vi "Teleop.vi"(10 "Match Info":T2={"Autonomous Elapsed Seconds"=0.0, "TeleOp Elapsed Seconds"=0.0, "Disabled Elapsed Seconds"=0.0, "Visited Autonomous"=FALSE, "Visited TeleOp"=FALSE, "Visited Disabled"=FALSE, "Autonomous Settings"={"Autonomous Style"=enum."Independent", "VI Refnum"=refnum}}, 11 "Call Context":T3) -> ()   [LabVIEW 2020]
doc: "This VI is called for each TeleOp packet received from the DS where the robot is not disabled. It is often used to read from the joysticks and update I/O or to update setpoints for timed control loops. It should complete and return within 20 milliseconds or it may miss DS packets."
uses:
  <vilib>/Rock Robotics/WPI/DriverStation/WPI_DriverStationDerivedRobotMode.ctl
  <vilib>/Rock Robotics/WPI/DriverStation/WPI_DriverStationMatch Info.ctl
  <vilib>/Rock Robotics/WPI/ThirdParty/Phoenix-LabVIEW/Motor Controller/Controls/CTRE_Phoenix_MotorControl_ControlMode.ctl
  <vilib>/Rock Robotics/Network Tables/NT Read Boolean.vi
  <vilib>/Rock Robotics/Network Tables/NT Read Number.vi
  <vilib>/Rock Robotics/WPI/ThirdParty/Phoenix-LabVIEW/CANCoder/Get/CTRE_Phoenix_CANcoder_GetSensorData.vi
  <vilib>/Rock Robotics/WPI/Utilities/WPI_GetSetVariantRefNum.vi
  <vilib>/addons/control/pid/pid.llb/PID (DBL).vi
  <vilib>/addons/control/pid/NI_PID_pid.lvlib
panel:
  in  "ScaleSpeed 4":dbl
  in  "ScaleSpeed 3":dbl
  in  "ScaleSpeed 2":dbl
  in  "ScaleSpeed":dbl
  in  "PID gains 2":T1={"proportional gain (Kc)"=0.002, "integral time (Ti, min)"=0.01, "derivative time (Td, min)"=0.0} {"derivative time (Td, min)" format="%.3f"; "integral time (Ti, min)" format="%.4f"; "proportional gain (Kc)" format="%.3f"}
  out "atan2(y,x)":dbl
  out "Absolute Position BL":dbl
  out "Absolute Position BR":dbl
  out "Absolute Position FL":dbl
  out "Absolute Position FR":dbl
  in  "PID gains":T1={"proportional gain (Kc)"=0.002, "integral time (Ti, min)"=0.01, "derivative time (Td, min)"=0.0} {"derivative time (Td, min)" format="%.3f"; "integral time (Ti, min)" format="%.4f"; "proportional gain (Kc)" format="%.3f"}
  in  "Output":dbl(knob) scale=-180.0..180.0
  out "Sample Slider 0":dbl(slide) scale=0.0..5.0
  out "Sample Boolean 1":bool
  out "Sample Boolean 0":bool
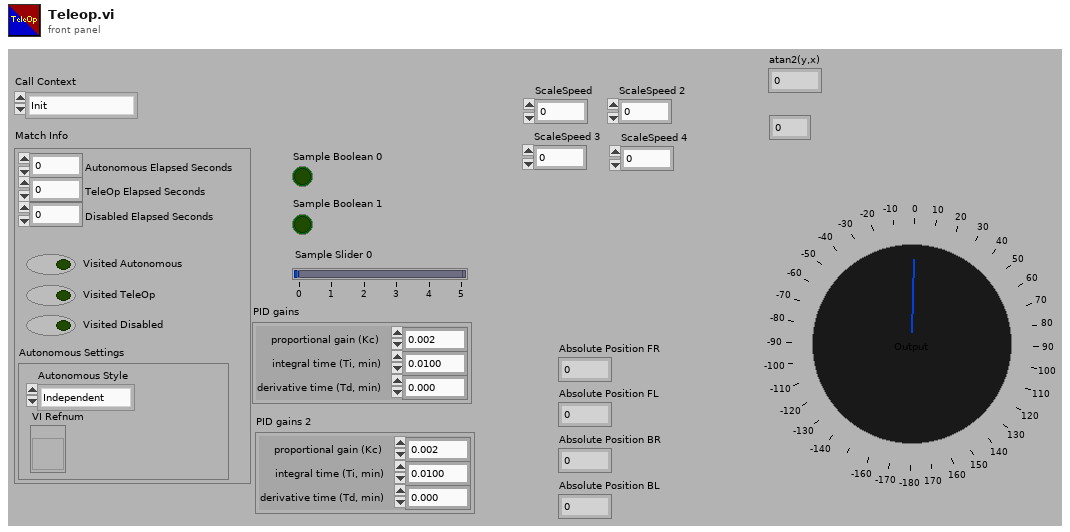
[diagram p1: front panel]
types:
  T1 = cluster{"proportional gain (Kc)":dbl, "integral time (Ti, min)":dbl, "derivative time (Td, min)":dbl}
  T2 = typedef "WPI_DriverStationMatch Info.ctl" = cluster{"Autonomous Elapsed Seconds":dbl, "TeleOp Elapsed Seconds":dbl, "Disabled Elapsed Seconds":dbl, "Visited Autonomous":bool, "Visited TeleOp":bool, "Visited Disabled":bool, "Autonomous Settings":cluster{"Autonomous Style":enum16{"Iterative", "Independent"}, "VI Refnum":refnum<vi>}}
  T3 = typedef "WPI_DriverStationDerivedRobotMode.ctl" = enum16{"Init", "Execute", "Stop"}
  T4 = typedef "CTRE_Phoenix_MotorControl_ControlMode.ctl" = u16
  T5 = typedef "CTRE_Phoenix_CANcoder_DeviceRef.ctl" = cluster{"DeviceStatus":errorcluster, "Device Number":u8, "Handle":u64, "UsageFrame":u32, "Library Path":path}
  T6 = typedef "WPI_JoystickDevRef.ctl" = cluster{"Device":T7}
  T7 = typedef "WPI_JoystickDeviceEnum.ctl" = enum16{"USB 0", "USB 1", "USB 2", "USB 3", "USB 4", "USB 5"}
  T8 = typedef "WPI_MotorControlDeviceRef.ctl" = cluster{"DeviceStatus":errorcluster, "Type":T9, "PWM":cluster{"PWM Channel":T10, "DeadBand":T11}, "CAN":cluster{"Device Number":u8, "SetOutput VI Ref":variant, "GetOutput VI Ref":variant, "Enable VI Ref":variant, "Disable VI Ref":variant, "Data":variant}, "Invert":bool, "DIO PWM":cluster{"PWM \"Enable\" Channel":T10, "DIOChannel":T12, "PWM Rate":dbl}}
  T9 = typedef "WPI_MotorControlType.ctl" = enum16{"PWM", "CAN", "DIO PWM"}
  T10 = typedef "FPGA_DIOPWMChannel.ctl" = enum8{"PWM 0", "PWM 1", "PWM 2", "PWM 3", "PWM 4", "PWM 5", "PWM 6", "PWM 7", "PWM 8", "PWM 9", "PWM MXP 0", "PWM MXP 1", "PWM MXP 2", "PWM MXP 3", "PWM MXP 4", "PWM MXP 5", "PWM MXP 6", "PWM MXP 7", "PWM MXP 8", "PWM MXP 9", "Invalid"}
  T11 = typedef "WPI_PWMDeadband.ctl" = cluster{"Name":string, "maxPositivePwm":i32, "minPositivePwm":i32, "centerPwm":i32, "maxNegativePwm":i32, "minNegativePwm":i32, "angularRange":u16}
  T12 = typedef "FPGA_DIOChannel.ctl" = enum8{"DIO 0", "DIO 1", "DIO 2", "DIO 3", "DIO 4", "DIO 5", "DIO 6", "DIO 7", "DIO 8", "DIO 9", "DIO MXP 0", "DIO MXP 1", "DIO MXP 2", "DIO MXP 3", "DIO MXP 4", "DIO MXP 5", "DIO MXP 6", "DIO MXP 7", "DIO MXP 8", "DIO MXP 9", "DIO MXP 10", "DIO MXP 11", "DIO MXP 12", "DIO MXP 13", "DIO MXP 14", "DIO MXP 15", "SPI Port CS1", "SPI Port CS2", "SPI Port CS3", "SPI Port MISO", "SPI Port MOSI", "Invalid"}
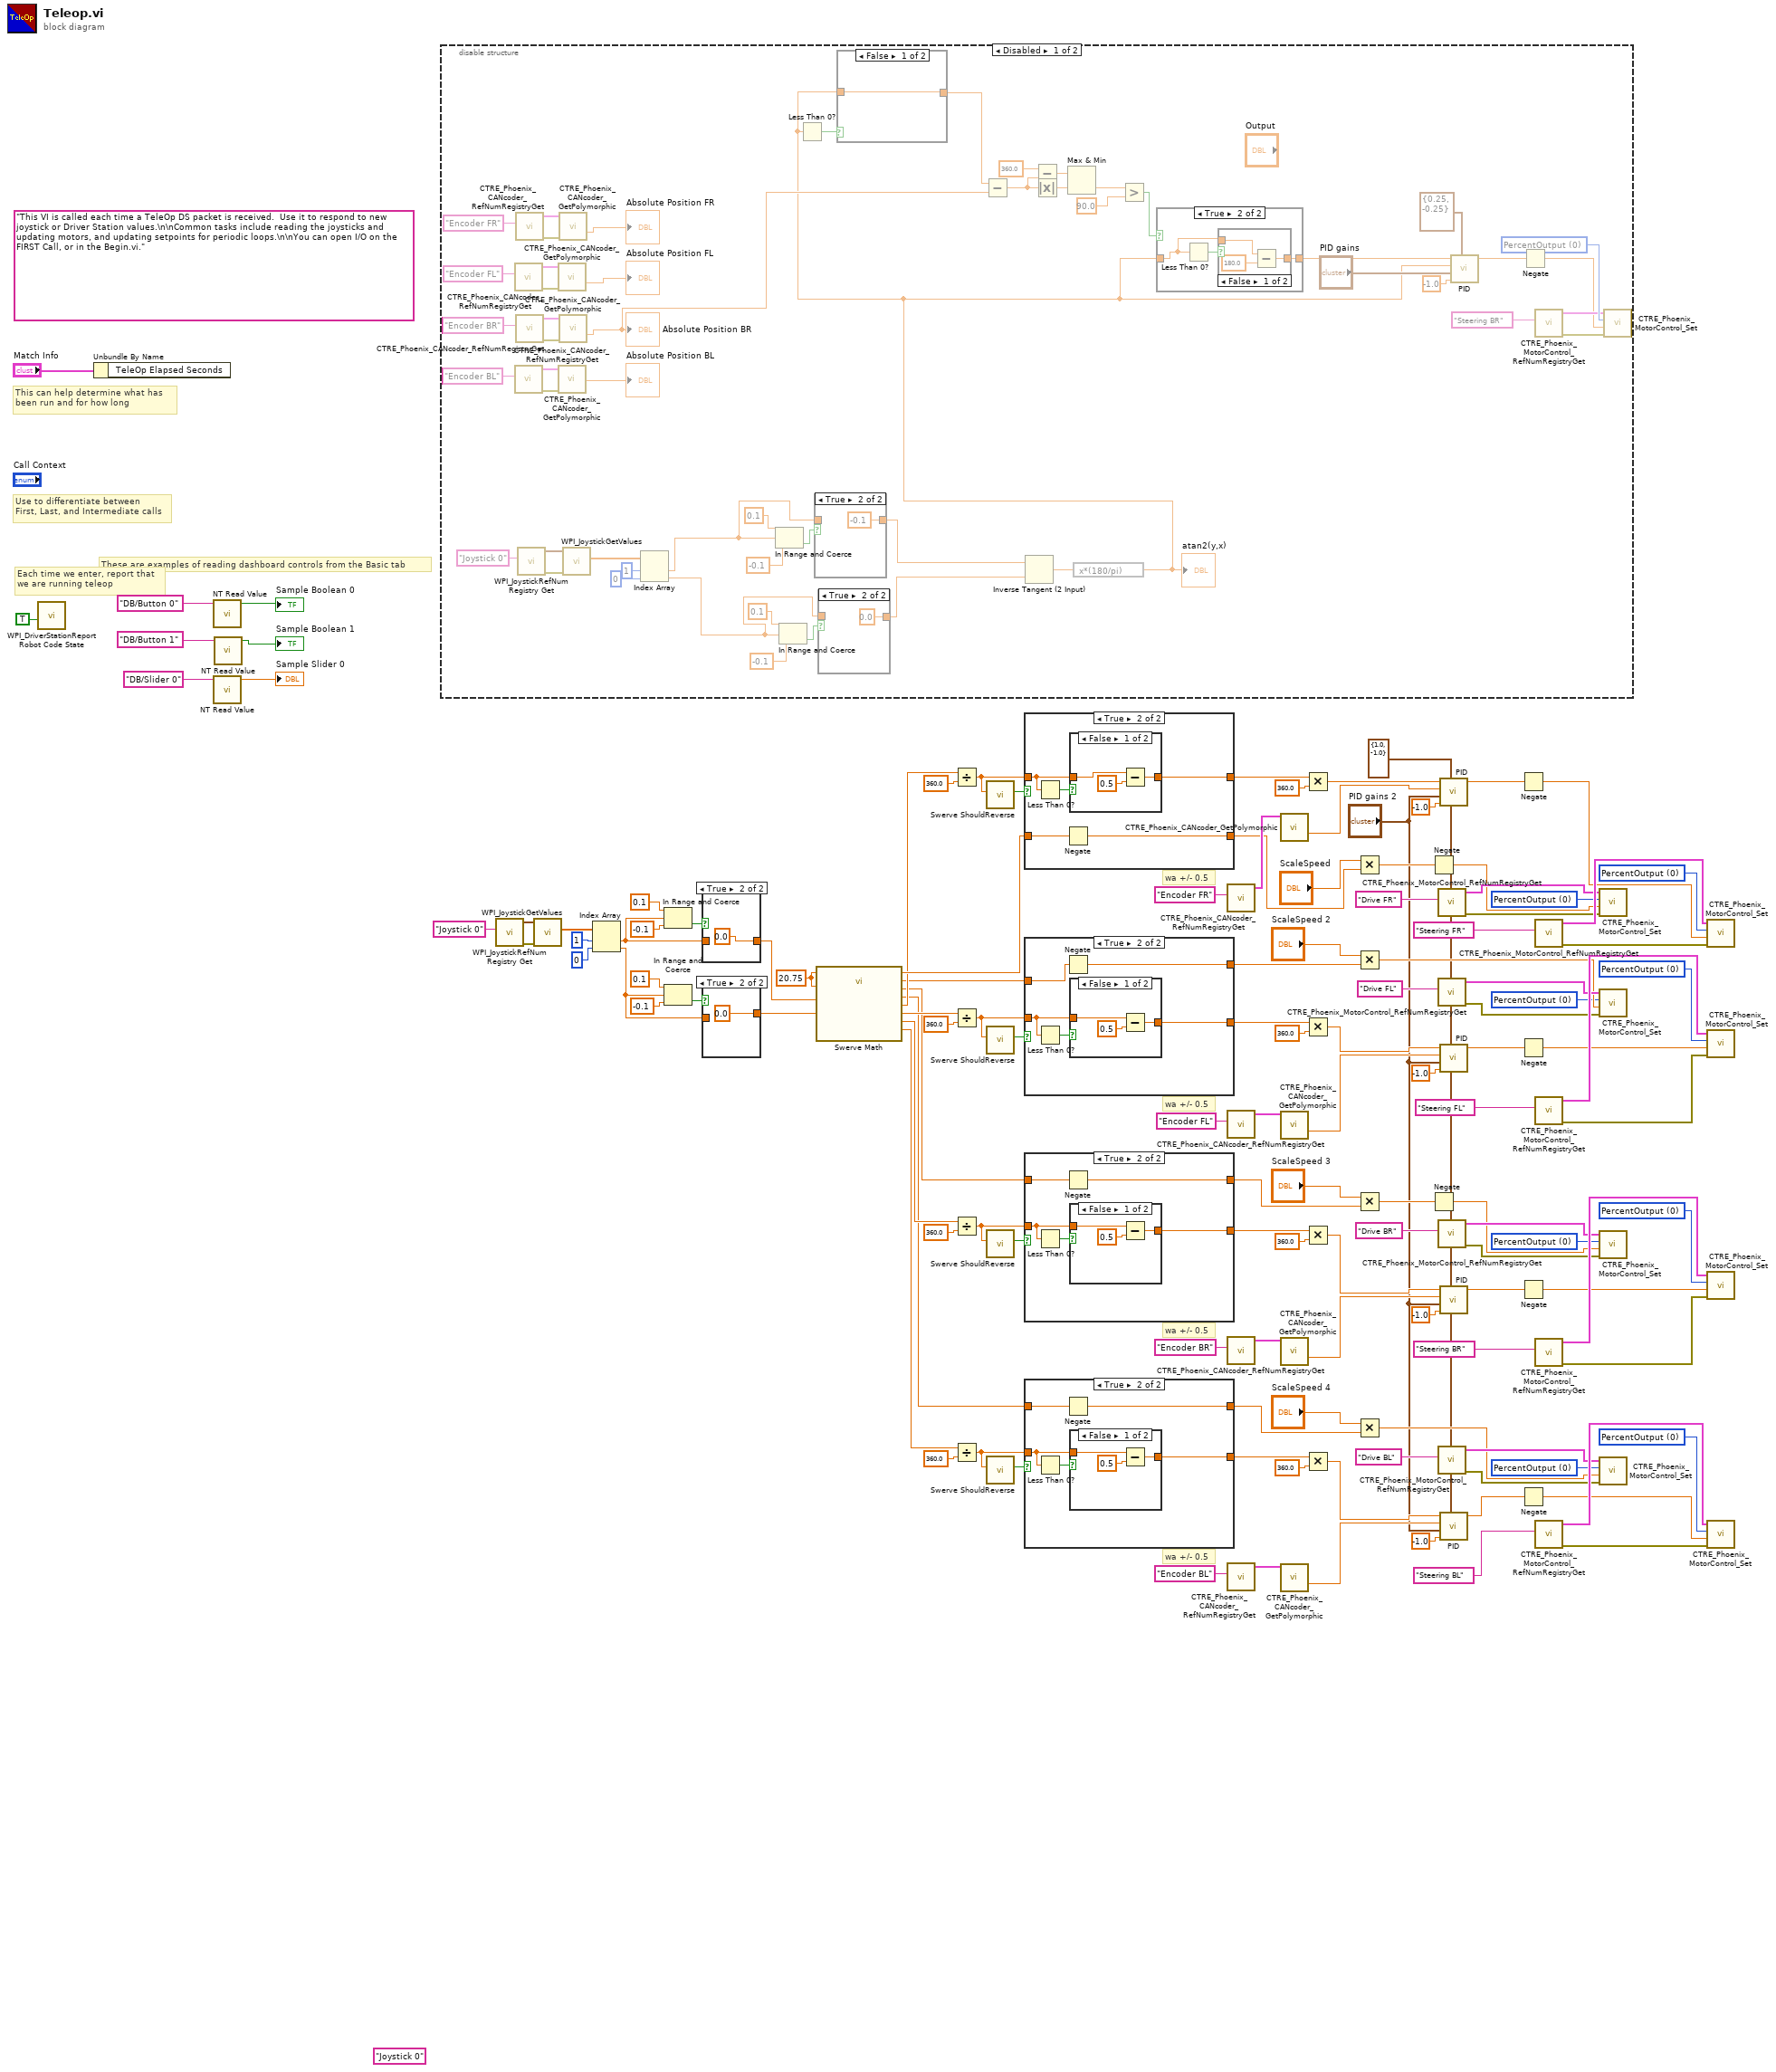
[diagram p0: block diagram]
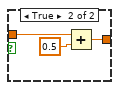
[diagram p3: hidden frame]
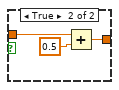
[diagram p5: hidden frame]
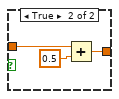
[diagram p7: hidden frame]
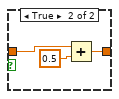
[diagram p9: hidden frame]
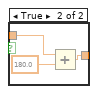
[diagram p13: hidden frame]
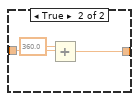
[diagram p14: hidden frame]
diagram:
  w12 = T4 0 items=["PercentOutput"=0, "Position"=1, "Velocity"=2, "Current"=3, "Follower"=5, "MotionProfile"=6, "MotionMagic"=7, "MotionProfileArc"=10, "Disabled"=15] ("Control Mode")
  (unwired) "Joystick 0" ("refnum name")
  w33 = T4 0 items=["PercentOutput"=0, "Position"=1, "Velocity"=2, "Current"=3, "Follower"=5, "MotionProfile"=6, "MotionMagic"=7, "MotionProfileArc"=10, "Disabled"=15] ("Control Mode")
  w35 = T4 0 items=["PercentOutput"=0, "Position"=1, "Velocity"=2, "Current"=3, "Follower"=5, "MotionProfile"=6, "MotionMagic"=7, "MotionProfileArc"=10, "Disabled"=15] ("Control Mode")
  w57 = T4 0 items=["PercentOutput"=0, "Position"=1, "Velocity"=2, "Current"=3, "Follower"=5, "MotionProfile"=6, "MotionMagic"=7, "MotionProfileArc"=10, "Disabled"=15] ("Control Mode")
  w58 = T4 0 items=["PercentOutput"=0, "Position"=1, "Velocity"=2, "Current"=3, "Follower"=5, "MotionProfile"=6, "MotionMagic"=7, "MotionProfileArc"=10, "Disabled"=15] ("Control Mode")
  w80 = T4 0 items=["PercentOutput"=0, "Position"=1, "Velocity"=2, "Current"=3, "Follower"=5, "MotionProfile"=6, "MotionMagic"=7, "MotionProfileArc"=10, "Disabled"=15] ("Control Mode")
  w82 = T4 0 items=["PercentOutput"=0, "Position"=1, "Velocity"=2, "Current"=3, "Follower"=5, "MotionProfile"=6, "MotionMagic"=7, "MotionProfileArc"=10, "Disabled"=15] ("Control Mode")
  w1 = cluster{"output high":dbl, "output low":dbl} {"output high"=1.0, "output low"=-1.0} ("output range")
  w120 = T4 0 items=["PercentOutput"=0, "Position"=1, "Velocity"=2, "Current"=3, "Follower"=5, "MotionProfile"=6, "MotionMagic"=7, "MotionProfileArc"=10, "Disabled"=15] ("Control Mode")
  w121 = 20.75 ("Trackwidth (W)")
  (unwired) "This VI is called each time a TeleOp DS packet is received.  Use it to respond to new joystick or Driver Station values.\n\nCommon tasks include reading the joysticks and updating motors, and updating setpoints for periodic loops.\n\nYou can open I/O on the FIRST Call, or in the Begin.vi."
  # "wa +/- 0.5"
  # "wa +/- 0.5"
  # "wa +/- 0.5"
  # "wa +/- 0.5"
  # "These are examples of reading dashboard controls from the Basic tab"
  # "Each time we enter, report that\nwe are running teleop"
  # "Use to differentiate between\nFirst, Last, and Intermediate calls"
  # "This can help determine what has\nbeen run and for how long"
  n1 = call <vilib>:"WPI_DriverStationReport Robot Code State.vi"("TeleOp"=TRUE ("Autonomous")) -> ()  [unwired: 10 in, 1 out]
  n2 = Unbundle By Name("Match Info") -> ()  [unwired: 1 out]
  n3 = call-poly <vilib>:"NT Read Value.vi"("Name"="DB/Button 0" ("refnum name")) -> ("Boolean"=→"Sample Boolean 0":bool)  [unwired: 9 in, 1 out]
  n4 = call-poly <vilib>:"NT Read Value.vi"("Name"="DB/Slider 0" ("refnum name")) -> ("Numeric"=→"Sample Slider 0":dbl)  [unwired: 9 in, 1 out]
  n5 = call-poly <vilib>:"NT Read Value.vi"("Name"="DB/Button 1" ("refnum name")) -> ("Boolean"=→"Sample Boolean 1":bool)  [unwired: 9 in, 1 out]
  n6 = disable-structure shown="Disabled" {
    frame Disabled {
      w165 = T4 0 items=["PercentOutput"=0, "Position"=1, "Velocity"=2, "Current"=3, "Follower"=5, "MotionProfile"=6, "MotionMagic"=7, "MotionProfileArc"=10, "Disabled"=15] ("Control Mode")
      n7 = call <vilib>:"CTRE_Phoenix_CANcoder_RefNumRegistryGet.vi"("refnum name"="Encoder FL") -> ("error out"=w153:errorcluster, "CTRE_CANcoder_DeviceRef"=w154:T5)  [unwired: 9 in]
      n8 = call <vilib>:"CTRE_Phoenix_CANcoder_RefNumRegistryGet.vi"("refnum name"="Encoder BL") -> ("error out"=w147:errorcluster, "CTRE_CANcoder_DeviceRef"=w148:T5)  [unwired: 9 in]
      n9 = call <vilib>:"CTRE_Phoenix_CANcoder_RefNumRegistryGet.vi"("refnum name"="Encoder FR") -> ("error out"=w156:errorcluster, "CTRE_CANcoder_DeviceRef"=w157:T5)  [unwired: 9 in]
      n10 = call <vilib>:"CTRE_Phoenix_CANcoder_RefNumRegistryGet.vi"("refnum name"="Encoder BR") -> ("error out"=w150:errorcluster, "CTRE_CANcoder_DeviceRef"=w151:T5)  [unwired: 9 in]
      n11 = call <vilib>:"WPI_JoystickRefNum Registry Get.vi"("refnum name"="Joystick 0") -> ("error out"=w182:errorcluster, "JoystickDevRef"=w181:T6)  [unwired: 9 in]
      n12 = call-poly <vilib>:"CTRE_Phoenix_CANcoder_GetPolymorphic.vi"("CTRE_CANcoder_DeviceRef"=w154, "error in"=w153) -> ("Absolute Position"=→"Absolute Position FL":dbl)  [unwired: 9 in, 4 out]
      n13 = call-poly <vilib>:"CTRE_Phoenix_CANcoder_GetPolymorphic.vi"("CTRE_CANcoder_DeviceRef"=w148, "error in"=w147) -> ("Absolute Position"=→"Absolute Position BL":dbl)  [unwired: 9 in, 4 out]
      n14 = call-poly <vilib>:"CTRE_Phoenix_CANcoder_GetPolymorphic.vi"("CTRE_CANcoder_DeviceRef"=w157, "error in"=w156) -> ("Absolute Position"=→"Absolute Position FR":dbl)  [unwired: 9 in, 4 out]
      n15 = call-poly <vilib>:"CTRE_Phoenix_CANcoder_GetPolymorphic.vi"("CTRE_CANcoder_DeviceRef"=w151, "error in"=w150) -> ("Absolute Position"=w132:dbl)  [unwired: 9 in, 4 out]
      "Absolute Position BR" <- w132
      n16 = call <vilib>:"WPI_JoystickGetValues.vi"("error in (no error)"=w182, "JoystickDevRef"=w181) -> ("Axes"=w179:dbl[])  [unwired: 5 in, 4 out]
      n17 = Index Array(array=w179, index #1=1 ("index"), index #2=0 ("index")) -> (element #1=w166:dbl, element #2=w167:dbl)
      n18 = In Range and Coerce(upper limit=0.1, x=w166, lower limit=-0.1) -> (In Range?=w173:bool)  [unwired: 1 out]
      n19 = In Range and Coerce(upper limit=0.1, x=w167, lower limit=-0.1) -> (In Range?=w172:bool)  [unwired: 1 out]
      n20 = case shown="True" w173 {
        tunnel: [w199 -0.1 ("upper limit")] -> w169
        tunnel: w166 -> [w199 _]
        frame False {
        }
        frame True {
        }
      }
      n21 = case shown="True" w172 {
        tunnel: [w197 0.0 ("upper limit")] -> w168
        tunnel: w167 -> [w197 _]
        frame False {
        }
        frame True {
        }
      }
      n22 = Inverse Tangent (2 Input)(1:w168, 2:w169) -> (0:w176:dbl)
      n23 = expression code="x*(180/pi)"(w176) -> (w130:dbl)
      "atan2(y,x)" <- w130
      n24 = Less Than 0?(x=w130) -> (x < 0?=w142:bool)
      n25 = case shown="False" w142 {
        tunnel: w130 -> [w193 w196]
        tunnel: [w193 w195] -> w141
        frame False {
        }
        frame True {
          n26 = Add(x=360.0, y=w196) -> (x+y=w195:dbl)
        }
      }
      n27 = Subtract(x=w141, y=w132) -> (x-y=w137:dbl)
      n28 = Subtract(x=360.0, y=w137) -> (x-y=w139:dbl)
      n29 = Absolute Value(x=w137) -> (abs(x)=w140:dbl)
      n30 = Max & Min(x=w139, y=w140) -> (min(x,y)=w136:dbl)  [unwired: 1 out]
      n31 = Greater?(x=w136, y=90.0) -> (0:w131:bool)
      n32 = case shown="True" w131 {
        tunnel: [w183 w186] -> w133
        tunnel: w130 -> [w183 w184]
        frame False {
        }
        frame True {
          n33 = Less Than 0?(x=w184) -> (x < 0?=w185:bool)
          n34 = case shown="False" w185 {
            tunnel: [w188 w191] -> w186
            tunnel: w184 -> [w187 w190]
            frame False {
              n35 = Subtract(x=w187, y=180.0) -> (x-y=w188:dbl)
            }
            frame True {
              n36 = Add(x=w190, y=180.0) -> (x+y=w191:dbl)
            }
          }
        }
      }
      n37 = call-poly <vilib>:"PID.vi"("output range"=cluster{"output high":dbl, "output low":dbl} {"output high"=0.25, "output low"=-0.25}, "dt (s)"=-1.0, "PID gains"="PID gains", "process variable"=w130, "setpoint"=w133) -> ("output"=w161:dbl)  [unwired: 5 in, 1 out]
      n38 = Negate(x=w161) -> (-x=w158:dbl)
      n39 = call <vilib>:"CTRE_Phoenix_MotorControl_RefNumRegistryGet.vi"("refnum name"="Steering BR") -> ("error out"=w163:errorcluster, "PhoenixMotorControlDevRef"=w164:T8)  [unwired: 9 in]
      n40 = call <vilib>:"CTRE_Phoenix_MotorControl_Set.vi"("error in (no error)"=w163, "Output"=w158, "Control Mode"=w165, "PhoenixMotorControlDevRef"=w164) -> ()  [unwired: 6 in, 2 out]
    }
    frame Enabled {
    }
  }
  n41 = call <vilib>:"WPI_JoystickRefNum Registry Get.vi"("refnum name"="Joystick 0") -> ("error out"=w112:errorcluster, "JoystickDevRef"=w111:T6)  [unwired: 9 in]
  n42 = call <vilib>:"WPI_JoystickGetValues.vi"("error in (no error)"=w112, "JoystickDevRef"=w111) -> ("Axes"=w109:dbl[])  [unwired: 5 in, 4 out]
  n43 = Index Array(array=w109, index #1=1 ("index"), index #2=0 ("index")) -> (element #1=w99:dbl, element #2=w100:dbl)
  n44 = In Range and Coerce(upper limit=0.1, x=w99, lower limit=-0.1) -> (In Range?=w104:bool)  [unwired: 1 out]
  n45 = In Range and Coerce(upper limit=0.1, x=w100, lower limit=-0.1) -> (In Range?=w103:bool)  [unwired: 1 out]
  n46 = case shown="True" w104 {
    tunnel: [w201 0.0 ("upper limit")] -> w97
    tunnel: w99 -> [w201 _]
    frame False {
    }
    frame True {
    }
  }
  n47 = case shown="True" w103 {
    tunnel: [w203 0.0 ("upper limit")] -> w98
    tunnel: w100 -> [w203 _]
    frame False {
    }
    frame True {
    }
  }
  n48 = call "Swerve Math.vi"("Trackwidth (W)"=w121, "Wheelbase (L)"=w121, "Y -FWD"=w97, "X1 STR"=w98) -> ("wa3"=w6:dbl, "wa4"=w4:dbl, "ws1"=w11:dbl, "ws2"=w9:dbl, "ws3"=w7:dbl, "ws4"=w5:dbl, "wa2"=w8:dbl, "wa1"=w10:dbl)  [unwired: 4 in]
  n49 = Divide(x=w10, y=360.0) -> (x/y=w93:dbl)
  n50 = Divide(x=w8, y=360.0) -> (x/y=w69:dbl)
  n51 = Divide(x=w6, y=360.0) -> (x/y=w46:dbl)
  n52 = Divide(x=w4, y=360.0) -> (x/y=w22:dbl)
  n53 = call "Swerve ShouldReverse.vi"("wa in"=w93) -> ("shouldReverse out"=w94:bool)  [unwired: 10 in]
  n54 = call "Swerve ShouldReverse.vi"("wa in"=w69) -> ("shouldReverse out"=w70:bool)  [unwired: 10 in]
  n55 = call "Swerve ShouldReverse.vi"("wa in"=w46) -> ("shouldReverse out"=w47:bool)  [unwired: 10 in]
  n56 = call "Swerve ShouldReverse.vi"("wa in"=w22) -> ("shouldReverse out"=w23:bool)  [unwired: 10 in]
  n57 = case shown="True" w94 {
    tunnel: w11 -> [w206 w207]
    tunnel: w93 -> [w205 w210]
    tunnel: [w206 w208] -> w92
    tunnel: [w205 w209] -> w90
    frame False {
    }
    frame True {
      n58 = Less Than 0?(x=w210) -> (x < 0?=w211:bool)
      n59 = Negate(x=w207) -> (-x=w208:dbl)
      n60 = case shown="False" w211 {
        tunnel: w210 -> [w213 w216]
        tunnel: [w212 w215] -> w209
        frame False {
          n61 = Subtract(x=w213, y=0.5) -> (x-y=w212:dbl)
        }
        frame True {
          n62 = Add(x=w216, y=0.5) -> (x+y=w215:dbl)
        }
      }
    }
  }
  n63 = case shown="True" w70 {
    tunnel: w9 -> [w219 w220]
    tunnel: w69 -> [w218 w223]
    tunnel: [w219 w221] -> w68
    tunnel: [w218 w222] -> w66
    frame False {
    }
    frame True {
      n64 = Less Than 0?(x=w223) -> (x < 0?=w224:bool)
      n65 = Negate(x=w220) -> (-x=w221:dbl)
      n66 = case shown="False" w224 {
        tunnel: w223 -> [w226 w229]
        tunnel: [w225 w228] -> w222
        frame False {
          n67 = Subtract(x=w226, y=0.5) -> (x-y=w225:dbl)
        }
        frame True {
          n68 = Add(x=w229, y=0.5) -> (x+y=w228:dbl)
        }
      }
    }
  }
  n69 = case shown="True" w47 {
    tunnel: w7 -> [w232 w233]
    tunnel: w46 -> [w231 w236]
    tunnel: [w232 w234] -> w45
    tunnel: [w231 w235] -> w43
    frame False {
    }
    frame True {
      n70 = Less Than 0?(x=w236) -> (x < 0?=w237:bool)
      n71 = Negate(x=w233) -> (-x=w234:dbl)
      n72 = case shown="False" w237 {
        tunnel: w236 -> [w239 w242]
        tunnel: [w238 w241] -> w235
        frame False {
          n73 = Subtract(x=w239, y=0.5) -> (x-y=w238:dbl)
        }
        frame True {
          n74 = Add(x=w242, y=0.5) -> (x+y=w241:dbl)
        }
      }
    }
  }
  n75 = case shown="True" w23 {
    tunnel: w5 -> [w245 w246]
    tunnel: w22 -> [w244 w249]
    tunnel: [w245 w247] -> w21
    tunnel: [w244 w248] -> w19
    frame False {
    }
    frame True {
      n76 = Less Than 0?(x=w249) -> (x < 0?=w250:bool)
      n77 = Negate(x=w246) -> (-x=w247:dbl)
      n78 = case shown="False" w250 {
        tunnel: w249 -> [w252 w255]
        tunnel: [w251 w254] -> w248
        frame False {
          n79 = Subtract(x=w252, y=0.5) -> (x-y=w251:dbl)
        }
        frame True {
          n80 = Add(x=w255, y=0.5) -> (x+y=w254:dbl)
        }
      }
    }
  }
  n81 = call <vilib>:"CTRE_Phoenix_CANcoder_RefNumRegistryGet.vi"("refnum name"="Encoder FR") -> ("CTRE_CANcoder_DeviceRef"=w114:T5)  [unwired: 9 in, 1 out]
  n82 = call <vilib>:"CTRE_Phoenix_CANcoder_RefNumRegistryGet.vi"("refnum name"="Encoder FL") -> ("CTRE_CANcoder_DeviceRef"=w74:T5)  [unwired: 9 in, 1 out]
  n83 = call <vilib>:"CTRE_Phoenix_CANcoder_RefNumRegistryGet.vi"("refnum name"="Encoder BR") -> ("CTRE_CANcoder_DeviceRef"=w51:T5)  [unwired: 9 in, 1 out]
  n84 = call <vilib>:"CTRE_Phoenix_CANcoder_RefNumRegistryGet.vi"("refnum name"="Encoder BL") -> ("CTRE_CANcoder_DeviceRef"=w27:T5)  [unwired: 9 in, 1 out]
  n85 = call-poly <vilib>:"CTRE_Phoenix_CANcoder_GetPolymorphic.vi"("CTRE_CANcoder_DeviceRef"=w114) -> ("Absolute Position"=w96:dbl)  [unwired: 10 in, 4 out]
  n86 = call-poly <vilib>:"CTRE_Phoenix_CANcoder_GetPolymorphic.vi"("CTRE_CANcoder_DeviceRef"=w74) -> ("Absolute Position"=w72:dbl)  [unwired: 10 in, 4 out]
  n87 = call-poly <vilib>:"CTRE_Phoenix_CANcoder_GetPolymorphic.vi"("CTRE_CANcoder_DeviceRef"=w51) -> ("Absolute Position"=w49:dbl)  [unwired: 10 in, 4 out]
  n88 = call-poly <vilib>:"CTRE_Phoenix_CANcoder_GetPolymorphic.vi"("CTRE_CANcoder_DeviceRef"=w27) -> ("Absolute Position"=w25:dbl)  [unwired: 10 in, 4 out]
  n89 = Multiply(x=w90, y=360.0) -> (x*y=w89:dbl)
  n90 = Multiply(x=w66, y=360.0) -> (x*y=w65:dbl)
  n91 = Multiply(x=w43, y=360.0) -> (x*y=w42:dbl)
  n92 = Multiply(x=w19, y=360.0) -> (x*y=w18:dbl)
  n93 = Multiply(x="ScaleSpeed", y=w92) -> (x*y=w83:dbl)
  n94 = Multiply(x="ScaleSpeed 2", y=w68) -> (x*y=w59:dbl)
  n95 = Multiply(x="ScaleSpeed 3", y=w45) -> (x*y=w36:dbl)
  n96 = Multiply(x="ScaleSpeed 4", y=w21) -> (x*y=w3:dbl)
  n97 = Negate(x=w83) -> (-x=w81:dbl)
  n98 = Negate(x=w36) -> (-x=w34:dbl)
  n99 = call <vilib>:"CTRE_Phoenix_MotorControl_RefNumRegistryGet.vi"("refnum name"="Drive FR") -> ("error out"=w85:errorcluster, "PhoenixMotorControlDevRef"=w86:T8)  [unwired: 9 in]
  n100 = call <vilib>:"CTRE_Phoenix_MotorControl_RefNumRegistryGet.vi"("refnum name"="Drive FL") -> ("error out"=w61:errorcluster, "PhoenixMotorControlDevRef"=w62:T8)  [unwired: 9 in]
  n101 = call <vilib>:"CTRE_Phoenix_MotorControl_RefNumRegistryGet.vi"("refnum name"="Drive BR") -> ("error out"=w38:errorcluster, "PhoenixMotorControlDevRef"=w39:T8)  [unwired: 9 in]
  n102 = call <vilib>:"CTRE_Phoenix_MotorControl_RefNumRegistryGet.vi"("refnum name"="Drive BL") -> ("error out"=w14:errorcluster, "PhoenixMotorControlDevRef"=w15:T8)  [unwired: 9 in]
  n103 = call-poly <vilib>:"PID.vi"("output range"=w1, "dt (s)"=-1.0, "PID gains"="PID gains 2", "process variable"=w96, "setpoint"=w89) -> ("output"=w116:dbl)  [unwired: 5 in, 1 out]
  n104 = call-poly <vilib>:"PID.vi"("output range"=w1, "dt (s)"=-1.0, "PID gains"="PID gains 2", "process variable"=w72, "setpoint"=w65) -> ("output"=w76:dbl)  [unwired: 5 in, 1 out]
  n105 = call-poly <vilib>:"PID.vi"("output range"=w1, "dt (s)"=-1.0, "PID gains"="PID gains 2", "process variable"=w49, "setpoint"=w42) -> ("output"=w53:dbl)  [unwired: 5 in, 1 out]
  n106 = call-poly <vilib>:"PID.vi"("output range"=w1, "dt (s)"=-1.0, "PID gains"="PID gains 2", "process variable"=w25, "setpoint"=w18) -> ("output"=w29:dbl)  [unwired: 5 in, 1 out]
  n107 = Negate(x=w116) -> (-x=w87:dbl)
  n108 = Negate(x=w76) -> (-x=w63:dbl)
  n109 = Negate(x=w53) -> (-x=w40:dbl)
  n110 = Negate(x=w29) -> (-x=w16:dbl)
  n111 = call <vilib>:"CTRE_Phoenix_MotorControl_RefNumRegistryGet.vi"("refnum name"="Steering FR") -> ("error out"=w118:errorcluster, "PhoenixMotorControlDevRef"=w119:T8)  [unwired: 9 in]
  n112 = call <vilib>:"CTRE_Phoenix_MotorControl_RefNumRegistryGet.vi"("refnum name"="Steering FL") -> ("error out"=w78:errorcluster, "PhoenixMotorControlDevRef"=w79:T8)  [unwired: 9 in]
  n113 = call <vilib>:"CTRE_Phoenix_MotorControl_RefNumRegistryGet.vi"("refnum name"="Steering BR") -> ("error out"=w55:errorcluster, "PhoenixMotorControlDevRef"=w56:T8)  [unwired: 9 in]
  n114 = call <vilib>:"CTRE_Phoenix_MotorControl_RefNumRegistryGet.vi"("refnum name"="Steering BL") -> ("error out"=w31:errorcluster, "PhoenixMotorControlDevRef"=w32:T8)  [unwired: 9 in]
  n115 = call <vilib>:"CTRE_Phoenix_MotorControl_Set.vi"("error in (no error)"=w85, "Output"=w81, "Control Mode"=w82, "PhoenixMotorControlDevRef"=w86) -> ()  [unwired: 6 in, 2 out]
  n116 = call <vilib>:"CTRE_Phoenix_MotorControl_Set.vi"("error in (no error)"=w61, "Output"=w59, "Control Mode"=w58, "PhoenixMotorControlDevRef"=w62) -> ()  [unwired: 6 in, 2 out]
  n117 = call <vilib>:"CTRE_Phoenix_MotorControl_Set.vi"("error in (no error)"=w38, "Output"=w34, "Control Mode"=w35, "PhoenixMotorControlDevRef"=w39) -> ()  [unwired: 6 in, 2 out]
  n118 = call <vilib>:"CTRE_Phoenix_MotorControl_Set.vi"("error in (no error)"=w14, "Output"=w3, "Control Mode"=w12, "PhoenixMotorControlDevRef"=w15) -> ()  [unwired: 6 in, 2 out]
  n119 = call <vilib>:"CTRE_Phoenix_MotorControl_Set.vi"("error in (no error)"=w118, "Output"=w87, "Control Mode"=w120, "PhoenixMotorControlDevRef"=w119) -> ()  [unwired: 6 in, 2 out]
  n120 = call <vilib>:"CTRE_Phoenix_MotorControl_Set.vi"("error in (no error)"=w78, "Output"=w63, "Control Mode"=w80, "PhoenixMotorControlDevRef"=w79) -> ()  [unwired: 6 in, 2 out]
  n121 = call <vilib>:"CTRE_Phoenix_MotorControl_Set.vi"("error in (no error)"=w55, "Output"=w40, "Control Mode"=w57, "PhoenixMotorControlDevRef"=w56) -> ()  [unwired: 6 in, 2 out]
  n122 = call <vilib>:"CTRE_Phoenix_MotorControl_Set.vi"("error in (no error)"=w31, "Output"=w16, "Control Mode"=w33, "PhoenixMotorControlDevRef"=w32) -> ()  [unwired: 6 in, 2 out]
